vi "RON.vi"(0 "System no.":i32=1 min=1 max=4 step=1, 2 "Axes to command":string[](array[string]), 3 "Reference mode":bool[](array[boolean]), 5 "error in":errorcluster, 6 "Without axis ID?":bool) -> (19 "error out":errorcluster)   [LabVIEW 2020]
doc: "Sets reference mode for given axes. If Without axis ID is TRUE, then Axes to command is ignored and first field of the Reference mode array is used for the reference mode.\nIf the reference mode of an axis is ON, the axis must be driven to the reference switch (using REF.vi or FRF.vi) or, if no reference switch is available, to a limit switch (positive limit switch: using MPL.vi or FPL.vi; negative limit switch: using MNL.vi or FNL.vi) before any other motion can be commanded in closed-loop operation.\nIf reference mode is OFF, no referencing is required for the axis. In closed-loop operation, only relative moves can be commanded (using MVR.vi), unless the actual position is set with POS.vi. Afterwards, relative and absolute moves can be commanded. \nFor stages with neither reference nor limit switch, reference mode is automatically OFF. \n\nWARNINGS: \nIf reference mode is switched off, and relative moves are commanded, stages can be driven into the mechanical hard stop if moving to a position which is outside the travel range!\nIf reference mode is switched off, and the actual position is incorrectly set with POS.vi, stages can be driven into the mechanical hard stop when moving to a position which is thought to be within the travel range of the stage, but actually is not.\n\nC-880K005: VI only supported when called through PI_Multix.vi\n\nE-712: Check HLP? answer to find out if RON is supported and E-712 user manual to find out for which type of stages RON can be used..\n\nAll other systems: Without axis ID = FALSE"
panel:
  # "Sets reference mode for given axes. If \"Without axis ID\" is\nTRUE, then \"Axes to command\" is ignored and first field of the \n\"Reference mode\" array is used for the reference mode."
  # "Warning: If reference mode is switched off, stages can be\ndriven into the mechanical hard stop. See manual for details."
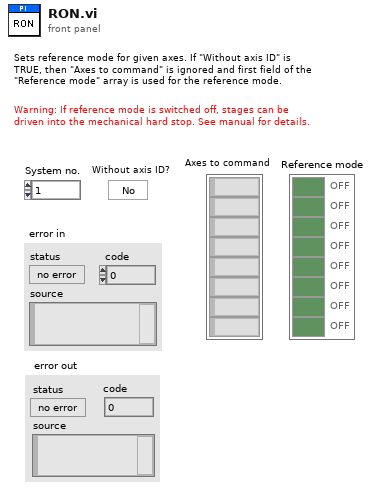
[diagram p1: front panel]
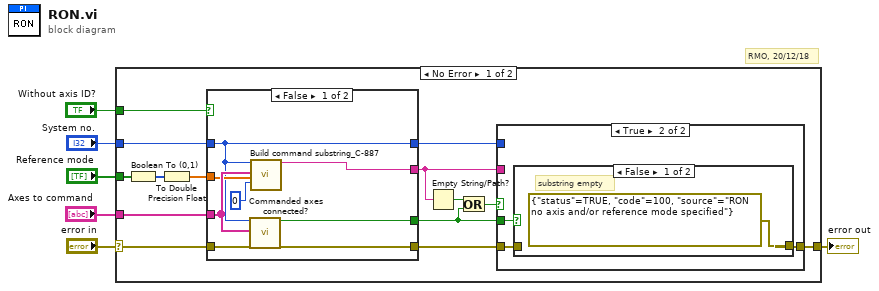
[diagram p0: block diagram]
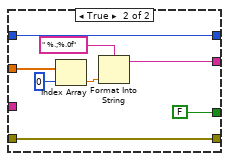
[diagram p2: hidden frame]
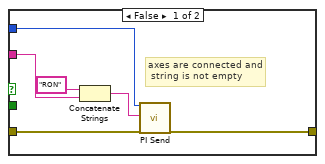
[diagram p3: hidden frame]
diagram:
  # "RMO, 20/12/18"
  n1 = case shown="No Error" "error in" {
    selector: "error in" -> [w13 w48]
    tunnel: [w20 w48] -> w6
    tunnel: "System no." -> [w8 _]
    tunnel: "Axes to command" -> [w18 _]
    tunnel: "Reference mode" -> [w17 _]
    tunnel: "Without axis ID?" -> [w14 _]
    frame No Error {
      n2 = Boolean To (0,1)(Boolean=w17) -> (0, 1=w16:i16[])
      n3 = To Double Precision Float(number=w16) -> (double precision float=w15:dbl[])
      n4 = case shown="False" w14 {
        tunnel: [w28 w30] -> w12
        tunnel: w13 -> [w27 w36]
        tunnel: [w26 w36] -> w19
        tunnel: w18 -> [w25 _]
        tunnel: [w24 FALSE] -> w10
        tunnel: w15 -> [w22 w33]
        tunnel: w8 -> [w21 w29]
        tunnel: [w21 w29] -> w7
        frame False {
          n5 = call "Commanded axes connected?.vi"("System no."=w21, "Commanded axes"=w25, "error in"=w27) -> ("Controller error"=w24:bool, "error out"=w26:errorcluster)  [unwired: 1 in, 14 out]
          n6 = call "Build command substring_C-887.vi"("System no."=w21, "Affected axes"=w25, "Parameters"=w22, "No. of digits"=i16 0 ("No.of digits")) -> ("Command substring"=w28:string)  [unwired: 3 in, 12 out]
        }
        frame True {
          n7 = Index Array(array=w33, index=0 ("Index")) -> (element=w32:dbl)
          n8 = Format Into String(format string=" %.;%.0f" ("Format String"), w32) -> (resulting string=w30:string)  [unwired: 2 in, 1 out]
        }
      }
      n9 = Empty String/Path?(string/path=w12) -> (empty?=w11:bool)
      n10 = Or(x=w11, y=w10) -> (x .or. y?=w9:bool)
      n11 = case shown="True" w9 {
        tunnel: w12 -> [w41 _]
        tunnel: [w38 w45] -> w20
        tunnel: w19 -> [w39 w43]
        tunnel: w10 -> [_ w44]
        tunnel: w7 -> [w37 _]
        frame False {
          # "axes are connected and\n string is not empty"
          n12 = Concatenate Strings("RON", w41) -> (w40:string)
          n13 = call "PI Send.vi"("System no."=w37, "String to send"=w40, "error in"=w39) -> ("error out"=w38:errorcluster)  [unwired: 3 in, 13 out]
        }
        frame True {
          # "substring empty or axis not connected"
          n14 = case shown="False" w44 {
            tunnel: [errorcluster {"status"=TRUE, "code"=100, "source"="RON no axis and/or reference mode specified"} ("error out") w47] -> w45
            tunnel: w43 -> [_ w47]
            frame False {
              # "substring empty"
            }
            frame True {
              # "commanded axis not connected"
            }
          }
        }
      }
    }
    frame Error {
    }
  }
  "error out" <- w6
